vi "Example StringName Increment.vi"() -> ()   [LabVIEW 2013]
uses:
  StringIncrement/StringIncrement.lvclass
  StringIncrement.Alphabetical/StringIncrement.Alphabetical.lvclass
panel:
  in  "Start":u32
  out "Result Strings":string[](array[string])
  in  "Input String":string="Filename"
  in  "Increment Function":enum16{"Numerical", "Alphabetical"}(ring)
  # "Modify the increment function to test \nNumerical representation vs Alphabetical representation"
  # "Change the start index for the increment."
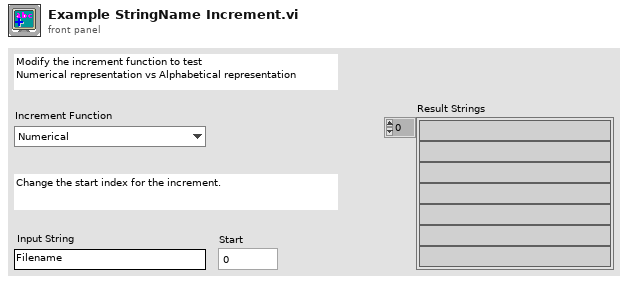
[diagram p1: front panel]
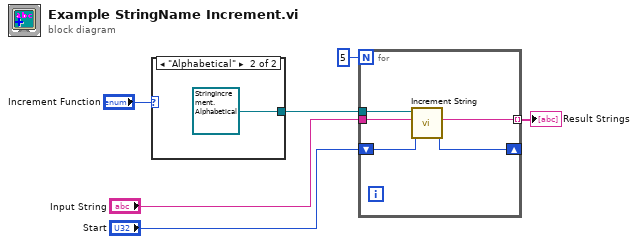
[diagram p0: block diagram]
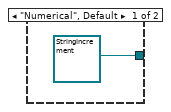
[diagram p2: hidden frame]
diagram:
  n1 = case shown="\"Alphabetical\"" "Increment Function" {
    tunnel: [refnum<class "StringIncrement.lvclass"> refnum ("StringIncrement.lvclass") refnum<class "StringIncrement.Alphabetical.lvclass"> refnum ("StringIncrement.Alphabetical.lvclass")] -> w5
    frame "Numerical", Default {
    }
    frame "Alphabetical" {
    }
  }
  n2 = for {
    N: 5 -> [_]
    tunnel: w5 -> [w13]
    tunnel: "Input String" -> [w12]
    shift-right: [w11] -> _
    shift-left: "Start" -> [w10]
    tunnel: [w9] -> w2 mode=indexing
    n3 = call "Increment String.vi"("Numeric"=w10, "Input String"=w12, "StringIncrement"=w13) -> ("Incremented Numeric"=w11:u32, "Incremented String"=w9:string)  [unwired: 7 in]
  }
  "Result Strings" <- w2
